vi "FSM Hunting.vi"(0 "Signals":T2, 2 "Detection Thr [%]":refnum<vi>, 3 "Manipulator Dynamics":refnum<vi>, 5 "Manipulator Controllers":T3, 7 "Sensed Resistance Levels":T1, 11 "error in (no error)":errorcluster, 13 "Dialog Indicator":refnum<vi>, 14 "Abort":refnum<vi>) -> (6 "Aborted":bool, 15 "error out":errorcluster)   [LabVIEW 2012, in "Autopatcher Daemon.lvlib"]
uses:
  Autopatcher Daemon.lvlib
  <vilib>/Analysis/baseanly.llb/Mean (DBL).vi
  <vilib>/Analysis/NI_AALBase.lvlib
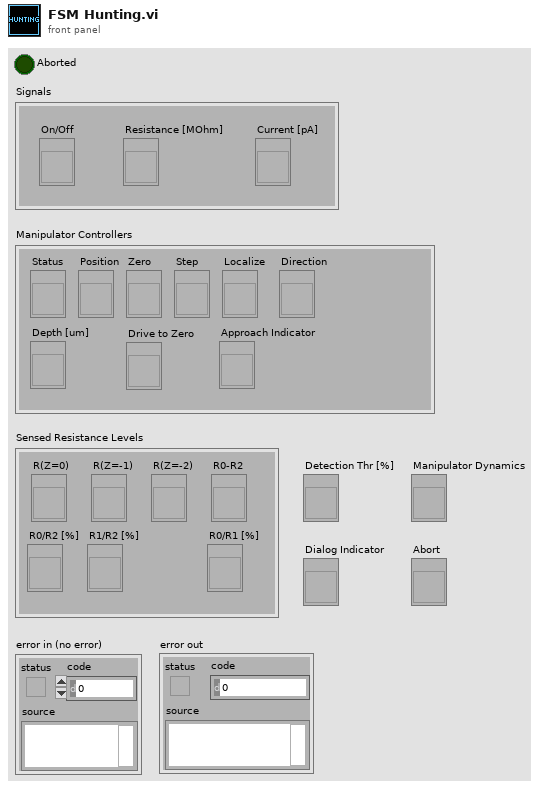
[diagram p1: front panel]
types:
  T1 = cluster{"R(Z=0)":refnum<vi>, "R(Z=-1)":refnum<vi>, "R(Z=-2)":refnum<vi>, "R0-R2":refnum<vi>, "R0/R2 [%]":refnum<vi>, "R1/R2 [%]":refnum<vi>, "R0/R1 [%]":refnum<vi>}
  T2 = cluster{"On/Off":refnum<vi>, "Resistance [MOhm]":refnum<vi>, "Current [pA]":refnum<vi>}
  T3 = cluster{"Status":refnum<vi>, "Position":refnum<vi>, "Zero":refnum<vi>, "Step":refnum<vi>, "Localize":refnum<vi>, "Approach Indicator":refnum<vi>, "Depth [um]":refnum<vi>, "Drive to Zero":refnum<vi>, "Direction":refnum<vi>}
  T4 = cluster{"Step length [um]":dbl, "Interstep Interval [ms]":u32, "Initial Speed [um/s]":dbl, "Max Speed [um/s]":dbl, "Acceleration [um/s^2]":dbl, "Max Depth [um]":dbl, "Max Penetration [um]":dbl}
  T5 = cluster{"X [um]":dbl, "Y [um]":dbl, "Z [um]":dbl}
  T6 = enum16{"Left Button", "Center Button", "Right Button", "Window Close"}
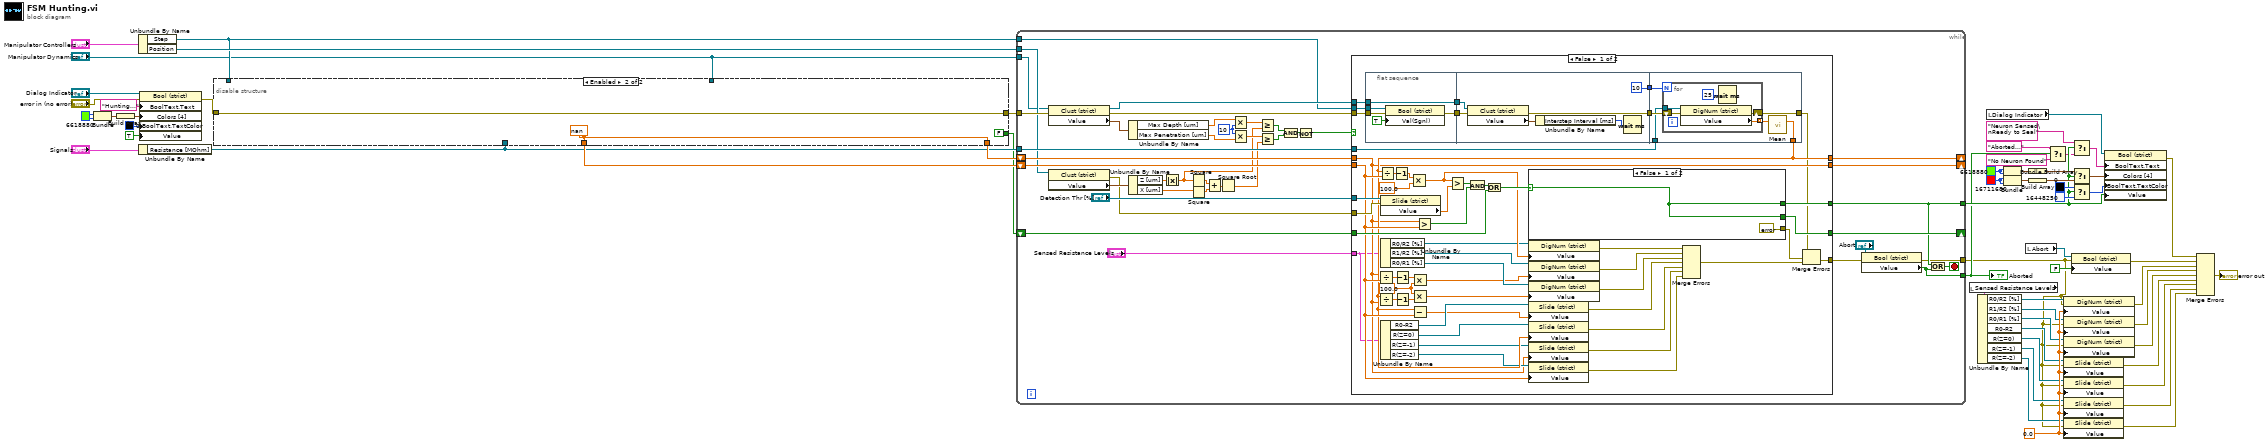
[diagram p0: block diagram]
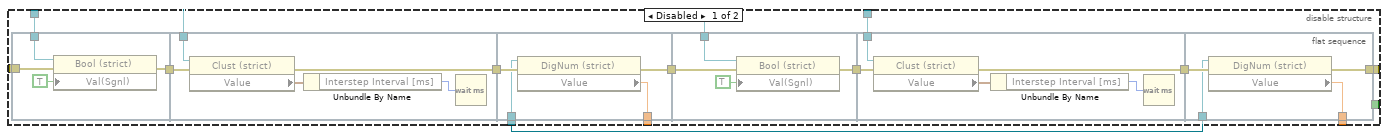
[diagram p2: hidden frame]
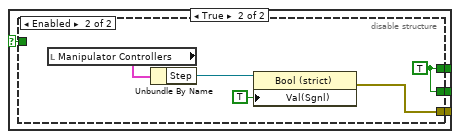
[diagram p3: hidden frame]
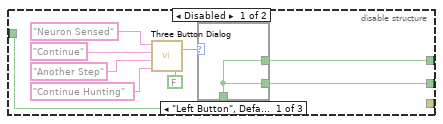
[diagram p4: hidden frame]
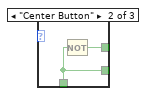
[diagram p5: hidden frame]
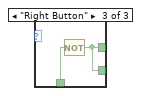
[diagram p6: hidden frame]
diagram:
  w17 = 0.0 ("Value")
  w27 = u32 6618880
  w48 = u32 16711680
  w51 = u32 6618880
  n1 = Bundle(w27, w27) -> (w32:cluster{u32, u32})  [unwired: 1 in]
  n2 = Build Array(w32) -> (w28:cluster{u32, u32}[])
  n3 = Unbundle By Name("Manipulator Controllers") -> ("Step"=w52:refnum<vi>, "Position"=w53:refnum<vi>)
  n4 = Unbundle By Name("Signals") -> ("Resistance [MOhm]"=w54:refnum<vi>)
  n5 = property class="Bool (strict)"(reference="Dialog Indicator", error in="error in (no error)", "BoolText.Text"="Hunting..." ("Boolean Text.Text"), "Colors [4]"=w28, "BoolText.TextColor"=u32 0, "Value"=TRUE) -> (error out=w24:errorcluster)  [unwired: 1 out]
  n6 = disable-structure shown="Enabled" {
    disable-tunnel: [w66 w99] -> w59
    disable-tunnel: [w65 w100] -> w58
    disable-tunnel: [w64 w100] -> w57
    disable-tunnel: w54 -> [w63 _]
    disable-tunnel: w52 -> [w62 _]
    disable-tunnel: "Manipulator Dynamics" -> [w61 _]
    disable-tunnel: w24 -> [w60 w99]
    disable-tunnel: [_ FALSE] -> w2
    frame Disabled {
      n7 = flat-sequence {
        tunnel: [w73] -> w71
        tunnel: w60 -> [w74]
        tunnel: w62 -> [w72]
        tunnel: w71 -> [w80]
        tunnel: [w79] -> w70
        tunnel: w61 -> [w76]
        tunnel: [w84] -> w65
        tunnel: [w82] -> w69
        tunnel: w70 -> [w83]
        tunnel: w63 -> [w81]
        tunnel: w69 -> [w87]
        tunnel: [w86] -> w68
        tunnel: w62 -> [w85]
        tunnel: w68 -> [w92]
        tunnel: [w91] -> w67
        tunnel: w61 -> [w89]
        tunnel: [w97] -> w64
        tunnel: [w95] -> w66
        tunnel: w67 -> [w96]
        tunnel: w63 -> [w94]
        frame #0 {
          n8 = property class="Bool (strict)"(reference=w72, error in=w74, "Val(Sgnl)"=TRUE ("Value (Signaling)")) -> (error out=w73:errorcluster)  [unwired: 1 out]
        }
        frame #1 {
          n9 = property class="Clust (strict)"(reference=w76, error in=w80) -> (error out=w79:errorcluster, "Value"=w78:T4)  [unwired: 1 out]
          n10 = Unbundle By Name(w78) -> ("Interstep Interval [ms]"=w77:u32)
          n11 = Wait (ms)(milliseconds to wait=w77) -> ()  [unwired: 1 out]
        }
        frame #2 {
          n12 = property class="DigNum (strict)"(reference=w81, error in=w83) -> (error out=w82:errorcluster, "Value"=w84:dbl)  [unwired: 1 out]
        }
        frame #3 {
          n13 = property class="Bool (strict)"(reference=w85, error in=w87, "Val(Sgnl)"=TRUE ("Value (Signaling)")) -> (error out=w86:errorcluster)  [unwired: 1 out]
        }
        frame #4 {
          n14 = property class="Clust (strict)"(reference=w89, error in=w92) -> (error out=w91:errorcluster, "Value"=w93:T4)  [unwired: 1 out]
          n15 = Unbundle By Name(w93) -> ("Interstep Interval [ms]"=w90:u32)
          n16 = Wait (ms)(milliseconds to wait=w90) -> ()  [unwired: 1 out]
        }
        frame #5 {
          n17 = property class="DigNum (strict)"(reference=w94, error in=w96) -> (error out=w95:errorcluster, "Value"=w97:dbl)  [unwired: 1 out]
        }
      }
    }
    frame Enabled {
      w100 = nan ("Value")
    }
  }
  n18 = while {
    tunnel: w59 -> [w113]
    tunnel: [w101] -> w1
    shift-right: [w138] -> _
    shift-left: w58 -> [w140]
    shift-right: [w137] -> _
    shift-left: w57 -> [w139]
    tunnel: [w104] -> w39
    shift-right: [w132] -> _
    shift-left: w2 -> [w133]
    tunnel: w54 -> [w126]
    tunnel: w53 -> [w111]
    tunnel: "Manipulator Dynamics" -> [w109]
    tunnel: w52 -> [w110]
    tunnel: [w103] -> w19
    stop <- w131 stop-if-true
    w129 = 10 ("y")
    n19 = property class="Clust (strict)"(reference=w109, error in=w113) -> (reference out=w112:refnum<vi>, error out=w125:errorcluster, "Value"=w130:T4)
    n20 = property class="Clust (strict)"(reference=w111) -> (error out=w105:errorcluster, "Value"=w115:T5)  [unwired: 1 in, 1 out]
    n21 = Unbundle By Name(w130) -> ("Max Depth [um]"=w128:dbl, "Max Penetration [um]"=w127:dbl)
    n22 = Unbundle By Name(w115) -> ("Z [um]"=w121:dbl, "X [um]"=w114:dbl)
    n23 = Absolute Value(x=w121) -> (abs(x)=w108:dbl)
    n24 = Square(x=w108) -> (x^2=w134:dbl)
    n25 = Square(x=w114) -> (x^2=w135:dbl)
    n26 = Add(x=w134, y=w135) -> (x+y=w136:dbl)
    n27 = Square Root(x=w136) -> (sqrt(x)=w120:dbl)
    n28 = Multiply(x=w128, y=w129) -> (x*y=w118:dbl)
    n29 = Multiply(x=w129, y=w127) -> (x*y=w119:dbl)
    n30 = Greater Or Equal?(x=w118, y=w108) -> (x >= y?=w123:bool)
    n31 = Greater Or Equal?(x=w119, y=w120) -> (x >= y?=w122:bool)
    n32 = Compound Arithmetic op=AND(w123, w122) -> (w117:bool)
    n33 = Not(x=w117) -> (.not. x?=w116:bool)
    n34 = case shown="False" w116 {
      selector: w116 -> [_ w240]
      tunnel: w125 -> [w192 w244]
      tunnel: [w148 w244] -> w102
      tunnel: w140 -> [w161 w243]
      tunnel: w139 -> [w154 w242]
      tunnel: [w154 w243] -> w138
      tunnel: [w159 w242] -> w137
      tunnel: [w187 w240] -> w104
      tunnel: w133 -> [w176 w241]
      tunnel: [w186 w241] -> w132
      tunnel: w112 -> [w182 _]
      tunnel: w126 -> [w180 _]
      tunnel: "Detection Thr [%]" -> [w179 _]
      tunnel: w105 -> [w175 _]
      tunnel: w110 -> [w174 _]
      tunnel: "Sensed Resistance Levels" -> [w147 _]
      frame False {
        w165 = 100.0 ("y")
        n35 = flat-sequence {
          tunnel: w192 -> [w219]
          tunnel: [w220] -> w191
          tunnel: w182 -> [w222]
          tunnel: [w222] -> w181
          tunnel: w174 -> [w218]
          tunnel: w191 -> [w228]
          tunnel: [w227] -> w183
          tunnel: w181 -> [w224]
          tunnel: [10] -> w143
          tunnel: [w229] -> w159
          tunnel: [w231] -> w142
          tunnel: w183 -> [w234]
          tunnel: w180 -> [w232]
          tunnel: w143 -> [w233]
          frame #0 {
            n36 = property class="Bool (strict)"(reference=w218, error in=w219, "Val(Sgnl)"=TRUE ("Value (Signaling)")) -> (error out=w220:errorcluster)  [unwired: 1 out]
          }
          frame #1 {
            n37 = property class="Clust (strict)"(reference=w224, error in=w228) -> (error out=w227:errorcluster, "Value"=w226:T4)  [unwired: 1 out]
            n38 = Unbundle By Name(w226) -> ("Interstep Interval [ms]"=w225:u32)
            n39 = Wait (ms)(milliseconds to wait=w225) -> ()  [unwired: 1 out]
          }
          frame #2 {
            n40 = for {
              N: w233 -> [_]
              tunnel: [w239] -> w230 mode=indexing
              tunnel: w232 -> [w237]
              shift-right: [w236] -> w231
              shift-left: w234 -> [w238]
              n41 = property class="DigNum (strict)"(reference=w237, error in=w238) -> (error out=w236:errorcluster, "Value"=w239:dbl)  [unwired: 1 out]
              n42 = Wait (ms)(milliseconds to wait=u32 25) -> ()  [unwired: 1 out]
            }
            n43 = call-poly <vilib>:"Mean.vi"("X"=w230) -> ("mean"=w229:dbl)  [unwired: 1 out]
          }
        }
        n44 = Divide(x=w154, y=w161) -> (x/y=w166:dbl)
        n45 = Divide(x=w159, y=w154) -> (x/y=w164:dbl)
        n46 = Divide(x=w159, y=w161) -> (x/y=w188:dbl)
        n47 = property class="Slide (strict)"(reference=w179, error in=w175) -> ("Value"=w178:dbl)  [unwired: 2 out]
        n48 = Unbundle By Name(w147) -> ("R0/R2 [%]"=w169:refnum<vi>, "R1/R2 [%]"=w168:refnum<vi>, "R0/R1 [%]"=w167:refnum<vi>)
        n49 = Unbundle By Name(w147) -> ("R0-R2"=w160:refnum<vi>, "R(Z=0)"=w155:refnum<vi>, "R(Z=-1)"=w158:refnum<vi>, "R(Z=-2)"=w157:refnum<vi>)
        n50 = Decrement(x=w188) -> (x-1=w144:dbl)
        n51 = Decrement(x=w166) -> (x-1=w146:dbl)
        n52 = Decrement(x=w164) -> (x-1=w145:dbl)
        n53 = Multiply(x=w144, y=100.0) -> (x*y=w170:dbl)
        n54 = Multiply(x=w146, y=w165) -> (x*y=w163:dbl)
        n55 = Multiply(x=w165, y=w145) -> (x*y=w162:dbl)
        n56 = Subtract(x=w159, y=w161) -> (x-y=w156:dbl)
        n57 = Greater?(x=w154, y=w161) -> (0:w177:bool)
        n58 = Greater?(x=w170, y=w178) -> (0:w190:bool)
        n59 = And(x=w190, y=w177) -> (x .and. y?=w184:bool)
        n60 = Or(x=w184, y=w176) -> (x .or. y?=w185:bool)
        n61 = case shown="False" w185 {
          selector: w185 -> [w194 w196]
          tunnel: [w194 w198] -> w187
          tunnel: [w194 w197] -> w186
          tunnel: [errorcluster {"status"=FALSE, "code"=0, "source"=""} ("error out") w195] -> w141
          frame False {
          }
          frame True {
            n62 = disable-structure shown="Enabled" {
              disable-tunnel: [w201 w217] -> w198
              disable-tunnel: [w200 w217] -> w197
              disable-tunnel: w196 -> [w199 _]
              disable-tunnel: [_ w215] -> w195
              frame Disabled {
                n63 = call <vilib>:"Three Button Dialog.vi"("Allow user to close window? (TRUE)"=FALSE, "Right Button Text (\"Cancel\")"="Continue Hunting" ("Right Button Text (\"Cancel\")"), "Center Button Text (\"No\")"="Another Step" ("Center Button Text (\"No\")"), "Left Button Text (\"Yes\")"="Continue" ("Left Button Text (\"Yes\")"), "message"="Neuron Sensed") -> ("Which Button?"=w202:T6)  [unwired: 6 in]
                n64 = case shown="\"Left Button\", Default" w202 {
                  tunnel: [w208 w210 w212] -> w201
                  tunnel: [w208 w209 w212] -> w200
                  tunnel: w199 -> [w208 w209 w211]
                  frame "Left Button", Default {
                  }
                  frame "Center Button" {
                    n65 = Not(x=w209) -> (.not. x?=w210:bool)
                  }
                  frame "Right Button" {
                    n66 = Not(x=w211) -> (.not. x?=w212:bool)
                  }
                }
              }
              frame Enabled {
                w217 = TRUE
                n67 = local read "Manipulator Controllers"() -> (w214:T3)
                n68 = Unbundle By Name(w214) -> ("Step"=w213:refnum<vi>)
                n69 = property class="Bool (strict)"(reference=w213, "Val(Sgnl)"=TRUE ("Value (Signaling)")) -> (error out=w215:errorcluster)  [unwired: 1 in, 1 out]
              }
            }
          }
        }
        n70 = property class="DigNum (strict)"(reference=w169, "Value"=w170) -> (error out=w151:errorcluster)  [unwired: 1 in, 1 out]
        n71 = property class="DigNum (strict)"(reference=w168, "Value"=w163) -> (error out=w152:errorcluster)  [unwired: 1 in, 1 out]
        n72 = property class="DigNum (strict)"(reference=w167, "Value"=w162) -> (error out=w153:errorcluster)  [unwired: 1 in, 1 out]
        n73 = property class="Slide (strict)"(reference=w160, "Value"=w156) -> (error out=w150:errorcluster)  [unwired: 1 in, 1 out]
        n74 = property class="Slide (strict)"(reference=w155, "Value"=w159) -> (error out=w173:errorcluster)  [unwired: 1 in, 1 out]
        n75 = property class="Slide (strict)"(reference=w158, "Value"=w154) -> (error out=w172:errorcluster)  [unwired: 1 in, 1 out]
        n76 = property class="Slide (strict)"(reference=w157, "Value"=w161) -> (error out=w171:errorcluster)  [unwired: 1 in, 1 out]
        n77 = Merge Errors(w151, w152, w153, w150, w173, w172, w171) -> (w149:errorcluster)
        n78 = Merge Errors(w142, w141, w149) -> (w148:errorcluster)
      }
      frame True {
      }
    }
    n79 = property class="Bool (strict)"(reference="Abort", error in=w102) -> (error out=w101:errorcluster, "Value"=w103:bool)  [unwired: 1 out]
    n80 = Or(x=w104, y=w103) -> (x .or. y?=w131:bool)
  }
  "Aborted" <- w19
  n81 = local read "Sensed Resistance Levels"() -> (w18:T1)
  n82 = Unbundle By Name(w18) -> ("R0/R2 [%]"=w16:refnum<vi>, "R1/R2 [%]"=w15:refnum<vi>, "R0/R1 [%]"=w14:refnum<vi>, "R0-R2"=w13:refnum<vi>, "R(Z=0)"=w12:refnum<vi>, "R(Z=-1)"=w11:refnum<vi>, "R(Z=-2)"=w10:refnum<vi>)
  n83 = local read "Dialog Indicator"() -> (w31:refnum<vi>)
  n84 = Bundle(w51, w51) -> (w50:cluster{u32, u32})  [unwired: 1 in]
  n85 = Bundle(w48, w48) -> (w47:cluster{u32, u32})  [unwired: 1 in]
  n86 = local read "Abort"() -> (w34:refnum<vi>)
  n87 = Build Array(w50) -> (w49:cluster{u32, u32}[])
  n88 = Build Array(w47) -> (w46:cluster{u32, u32}[])
  n89 = Select(t="Aborted...", s=w19, f="No Neuron Found" ("Boolean Text.Text")) -> (s? t:f=w22:string)
  n90 = property class="DigNum (strict)"(reference=w16, error in=w1, "Value"=w17) -> (error out=w9:errorcluster)  [unwired: 1 out]
  n91 = property class="DigNum (strict)"(reference=w15, error in=w1, "Value"=w17) -> (error out=w8:errorcluster)  [unwired: 1 out]
  n92 = property class="DigNum (strict)"(reference=w14, error in=w1, "Value"=w17) -> (error out=w7:errorcluster)  [unwired: 1 out]
  n93 = property class="Slide (strict)"(reference=w13, error in=w1, "Value"=w17) -> (error out=w6:errorcluster)  [unwired: 1 out]
  n94 = property class="Slide (strict)"(reference=w12, error in=w1, "Value"=w17) -> (error out=w5:errorcluster)  [unwired: 1 out]
  n95 = property class="Slide (strict)"(reference=w11, error in=w1, "Value"=w17) -> (error out=w4:errorcluster)  [unwired: 1 out]
  n96 = property class="Slide (strict)"(reference=w10, error in=w1, "Value"=w17) -> (error out=w3:errorcluster)  [unwired: 1 out]
  n97 = property class="Bool (strict)"(reference=w34, error in=w1, "Value"=FALSE) -> (error out=w38:errorcluster)  [unwired: 1 out]
  n98 = Select(t="Neuron Sensed\nReady to Seal" ("Boolean Text.Text"), s=w39, f=w22) -> (s? t:f=w43:string)
  n99 = Select(t=w49, s=w39, f=w46) -> (s? t:f=w44:cluster{u32, u32}[])
  n100 = Select(t=u32 0, s=w39, f=u32 16448250) -> (s? t:f=w40:u32)
  n101 = property class="Bool (strict)"(reference=w31, "BoolText.Text"=w43, "Colors [4]"=w44, "BoolText.TextColor"=w40, "Value"=w39) -> (error out=w37:errorcluster)  [unwired: 1 in, 1 out]
  n102 = Merge Errors(w37, w38, w9, w8, w7, w6, w5, w4, w3) -> (→"error out":errorcluster)
